vi "Sequencer Main.vi"() -> ()   [LabVIEW 2018] (continued)
                                frame True {
                                n2569 = Scan From String(format string="%d", input string=w5408, initial scan location=u32 1) -> (output 1=w5405:i32)  [unwired: 2 in, 3 out]
                                }
                                }
                                n2570 = In Range and Coerce(upper limit=w5398, x=w5395, lower limit=w5397) -> (In Range?=w5396:bool)  [unwired: 1 out]
                                }
                                }
                                n2571 = Replace Array Subset(array=w5392, new element=w5388, index=3) -> (w5391:errorcluster[])
                                n2572 = global write "Global Variable.vi" "Array Errors"(w5391) -> ()
                                n2573 = Number To Decimal String(number=w5383) -> (decimal integer string=w5371:string)  [unwired: 1 in]
                                n2574 = Concatenate Strings(w5378, "::") -> (w5379:string)
                                n2575 = Concatenate Strings(w5382, w5381, w5382, w5379, w5374, w5375, w5373, w5374, w5371, w5373, w5374, w5372, w5373, w5380, w5381, w5380) -> (w5376:string)
                                n2576 = case shown="False" w5384 {
                                tunnel: [enum16{"Idle", "PASS", "FALSE"}."FALSE" ("Step Test Result") enum16{"Idle", "PASS", "FALSE"}."PASS" ("Step Test Result")] -> w5389
                                frame False {
                                # "Step TEST Result"
                                }
                                frame True {
                                # "Step TEST Result"
                                }
                                }
                                n2577 = invoke on="Serial CMD Mon" class="Str" method="Append String"("string"=w5376) -> ()  [unwired: 3 in, 4 out]
                                }
                                frame #2 {
                                }
                              }
                              n2578 = global read "Global Variable.vi" "Array_Measurement"() -> (w5339:dbl[])
                              n2579 = Decimal String To Number(string=w5329) -> (number=w5340:i32)  [unwired: 2 in, 1 out]
                              n2580 = Index Array(array=w5339, index=w5340) -> (element=w5338:dbl)
                              n2581 = in-place {
                                in-place-border: w5338 -> [w5358]
                                in-place-border: [w5356] -> w5337
                                in-place-border: [w5353] -> w5336
                                w5354 = 1000.0 ("y")
                                # "Calculate +-3%"
                                n2582 = Multiply(x=w5358, y=1.03) -> (x*y=w5359:dbl)
                                n2583 = Multiply(x=w5358, y=0.97) -> (x*y=w5355:dbl)
                                n2584 = Multiply(x=w5359, y=w5354) -> (x*y=w5356:dbl)
                                n2585 = Multiply(x=w5354, y=w5355) -> (x*y=w5353:dbl)
                              }
                              n2586 = To Unsigned Long Integer(number=w5337) -> (unsigned 32bit integer=w5334:u32)
                              n2587 = To Unsigned Long Integer(number=w5336) -> (unsigned 32bit integer=w5335:u32)
                              n2588 = Number To Decimal String(number=w5334) -> (decimal integer string=w5332:string)  [unwired: 1 in]
                              n2589 = Number To Decimal String(number=w5335) -> (decimal integer string=w5330:string)  [unwired: 1 in]
                              n2590 = Concatenate Strings("max " ("string"), w5332) -> (w5324:string)
                              n2591 = Concatenate Strings("min " ("string"), w5330) -> (w5323:string)
                              n2592 = Concatenate Strings(w5324, "\r\n", w5323) -> (w5325:string)
                              n2593 = in-place {
                                in-place-border: w5327 -> [w5348]
                                in-place-border: w5325 -> [w5346]
                                # "Set Parameters to \nTest Seguenser Table"
                                n2594 = global read "Global Variable.vi" "Current Step Nmb"() -> (w5350:u32)
                                n2595 = property on="Test Squencer Edit" class="MCListbox (strict)"() -> ("ItemNames"=w5352:string[][])  [unwired: 2 in, 2 out]
                                n2596 = Replace Array Subset(array=w5352, new element #1=w5348, index (row) #1=w5350, index (col) #1=2 ("disabled index (col)"), new element #2=w5346, index (row) #2=w5350, index (col) #2=4 ("disabled index (col)")) -> (w5351:string[][])
                                n2597 = property on="Test Squencer Edit" class="MCListbox (strict)"("ItemNames"=w5351) -> ()  [unwired: 2 in, 2 out]
                              }
                            }
                            frame "capmem" {
                              w5419 = "max: "
                              w5420 = ">" ("string")
                              w5422 = "<" ("string")
                              w5424 = "min: "
                              # "Parameters"
                              # "Cmd"
                              n2598 = flat-sequence {
                                tunnel: [w5456] -> w5442
                                tunnel: [w5455] -> w5441
                                tunnel: [w5454] -> w5413
                                tunnel: w5442 -> [w5491]
                                tunnel: w5441 -> [w5492]
                                tunnel: w5438 -> [w5490]
                                tunnel: w5433 -> [w5489]
                                tunnel: w5437 -> [w5487]
                                tunnel: w5436 -> [w5486]
                                tunnel: [w5485] -> w5429
                                tunnel: [w5488] -> w5415
                                tunnel: [w5569] -> w5414
                                tunnel: w5415 -> [w5569]
                                frame #0 {
                                n2599 = for {
                                N: 1 -> [_]
                                tunnel: [w5461] -> w5456
                                tunnel: [w5460] -> w5455
                                tunnel: [w5458] -> w5454
                                i -> [w5459]
                                n2600 = case shown="1" w5459 {
                                tunnel: [w5467 w5481] -> w5461
                                tunnel: [w5463 w5474] -> w5460
                                tunnel: [w5462 w5473] -> w5458
                                frame 0, Default {
                                n2601 = global read "Global Variable.vi" "COM Port FTDI RS232"() -> (w5470:refnum<visa-resource-name>)
                                n2602 = call "ADB-Serial_WrRd.vi"("Timeout(Sec)"=2.0, "PassString"="Chuck(3)", "Command"="capmem 1", "ComPort"=w5470) -> ("error out"=w5464:errorcluster, "PASS"=w5467:bool, "received"=w5462:string)  [unwired: 5 in]
                                n2603 = invoke on="Serial CMD Mon" class="Str" method="Append String"(error in=w5464, "string"=w5462) -> (error out=w5463:errorcluster)  [unwired: 2 in, 3 out]
                                n2604 = Wait (ms)(milliseconds to wait=u32 1000) -> ()  [unwired: 1 out]
                                }
                                frame 1 {
                                w5471 = u16 2 items=["None", "XON/XOFF", "RTS/CTS", "XON/XOFF & RTS/CTS", "DTR/DSR", "XON/XOFF & DTR/DSR"] ("flow control (0:none)")
                                w5476 = "\r\n"
                                n2605 = global read "Global Variable.vi" "COM Port FTDI RS232"() -> (w5484:refnum<visa-resource-name>)
                                n2606 = call "ADB-Serial_WrRd.vi"("flow control (0:none)"=w5471, "Tx Deay"=u16 5, "Timeout(Sec)"=2.0, "PassString"="Chuck(3)", "Command"="capmem 0", "ComPort"=w5484) -> ("error out"=w5475:errorcluster, "PASS"=w5481:bool, "received"=w5473:string)  [unwired: 3 in]
                                n2607 = Concatenate Strings(w5473, w5476, "DELAY->5Sec", w5476) -> (w5478:string)
                                n2608 = invoke on="Serial CMD Mon" class="Str" method="Append String"(error in=w5475, "string"=w5478) -> (error out=w5474:errorcluster)  [unwired: 2 in, 3 out]
                                n2609 = Wait (ms)(milliseconds to wait=u32 4500) -> ()  [unwired: 1 out]
                                }
                                }
                                }
                                }
                                frame #1 {
                                n2610 = case shown="True" w5491 {
                                tunnel: w5490 -> [_ w5509]
                                tunnel: w5489 -> [_ w5508]
                                tunnel: [enum16{"Idle", "PASS", "FALSE"}."FALSE" ("Step Test Result") w5507] -> w5488
                                tunnel: w5487 -> [_ w5506]
                                tunnel: w5486 -> [_ w5505]
                                tunnel: [i32[] [0, 0] w5498] -> w5485
                                frame False {
                                }
                                frame True {
                                n2611 = for {
                                N: 2 -> [_]
                                tunnel: w5509 -> [w5518]
                                tunnel: w5508 -> [w5517]
                                tunnel: w5506 -> [w5516]
                                tunnel: w5505 -> [w5515]
                                tunnel: [w5514] -> w5504 mode=indexing
                                tunnel: [w5513] -> w5498 mode=indexing
                                i -> [w5519]
                                n2612 = case shown="1" w5519 {
                                tunnel: w5518 -> [w5534 _]
                                tunnel: w5517 -> [w5533 _]
                                tunnel: w5516 -> [_ w5553]
                                tunnel: w5515 -> [_ w5552]
                                tunnel: [w5527 w5551] -> w5514
                                tunnel: [w5520 w5547] -> w5513
                                frame 0, Default {
                                w5523 = "\r\n"
                                n2613 = global read "Global Variable.vi" "COM Port FTDI RS232"() -> (w5540:refnum<visa-resource-name>)
                                n2614 = Wait (ms)(milliseconds to wait=u32 4500) -> ()  [unwired: 1 out]
                                n2615 = call "ADB-Serial_WrRd.vi"("Timeout(Sec)"=3.0, "PassString"="Chuck(3)", "Command"="capmem", "ComPort"=w5540) -> ("error out"=w5522:errorcluster, "PASS"=w5528:bool, "received"=w5525:string)  [unwired: 5 in]
                                n2616 = property on="Msg Str" class="Str"("Text.Scroll Position"=inf) -> ()  [unwired: 2 in, 2 out]
                                n2617 = Match Pattern(string=w5525, regular expression="voltage") -> (after substring=w5538:string)  [unwired: 1 in, 3 out]
                                n2618 = Concatenate Strings(w5525, w5523, "DELAY->5Sec", w5523) -> (w5526:string)
                                n2619 = Scan From String(format string="%d", input string=w5538, initial scan location=u32 0) -> (output 1=w5520:i32)  [unwired: 2 in, 3 out]
                                n2620 = global read "Global Variable.vi" "Array Errors"() -> (w5530:errorcluster[])
                                n2621 = In Range and Coerce(upper limit=w5534, x=w5520, lower limit=w5533) -> (In Range?=w5529:bool)  [unwired: 1 out]
                                n2622 = invoke on="Serial CMD Mon" class="Str" method="Append String"(error in=w5522, "string"=w5526) -> (error out=w5521:errorcluster)  [unwired: 2 in, 3 out]
                                n2623 = Replace Array Subset(array=w5530, new element=w5521, index=3) -> (w5531:errorcluster[])
                                n2624 = And(x=w5529, y=w5528) -> (x .and. y?=w5527:bool)
                                n2625 = global write "Global Variable.vi" "Array Errors"(w5531) -> ()
                                }
                                frame 1 {
                                w5545 = u16 2 items=["None", "XON/XOFF", "RTS/CTS", "XON/XOFF & RTS/CTS", "DTR/DSR", "XON/XOFF & DTR/DSR"] ("flow control (0:none)")
                                n2626 = global read "Global Variable.vi" "COM Port FTDI RS232"() -> (w5564:refnum<visa-resource-name>)
                                n2627 = call "ADB-Serial_WrRd.vi"("flow control (0:none)"=w5545, "Tx Deay"=u16 5, "Timeout(Sec)"=3.0, "PassString"="Chuck(3)", "Command"="capmem", "ComPort"=w5564) -> ("error out"=w5549:errorcluster, "PASS"=w5554:bool, "received"=w5550:string)  [unwired: 3 in]
                                n2628 = invoke on="Serial CMD Mon" class="Str" method="Append String"("string"=w5550) -> ()  [unwired: 3 in, 4 out]
                                n2629 = property on="Msg Str" class="Str"(error in=w5549, "Text.Scroll Position"=inf) -> (error out=w5548:errorcluster)  [unwired: 1 in, 1 out]
                                n2630 = Match Pattern(string=w5550, regular expression="voltage") -> (after substring=w5562:string)  [unwired: 1 in, 3 out]
                                n2631 = Scan From String(format string="%d", input string=w5562, initial scan location=u32 0) -> (output 1=w5547:i32)  [unwired: 2 in, 3 out]
                                n2632 = global read "Global Variable.vi" "Array Errors"() -> (w5556:errorcluster[])
                                n2633 = In Range and Coerce(upper limit=w5553, x=w5547, lower limit=w5552) -> (In Range?=w5555:bool)  [unwired: 1 out]
                                n2634 = Replace Array Subset(array=w5556, new element=w5548, index=3) -> (w5557:errorcluster[])
                                n2635 = global write "Global Variable.vi" "Array Errors"(w5557) -> ()
                                n2636 = And(x=w5555, y=w5554) -> (x .and. y?=w5551:bool)
                                n2637 = Wait (ms)(milliseconds to wait=u32 1000) -> ()  [unwired: 1 out]
                                }
                                }
                                }
                                n2638 = Index Array(array=w5504, index #1=0 ("index"), index #2=1 ("index")) -> (element #1=w5503:bool, element #2=w5502:bool)
                                n2639 = And(x=w5503, y=w5502) -> (x .and. y?=w5501:bool)
                                n2640 = case shown="True" w5501 {
                                tunnel: [enum16{"Idle", "PASS", "FALSE"}."FALSE" ("Step Test Result") enum16{"Idle", "PASS", "FALSE"}."PASS" ("Step Test Result")] -> w5507
                                frame False {
                                # "Step TEST Result"
                                }
                                frame True {
                                # "Step TEST Result"
                                }
                                }
                                }
                                }
                                n2641 = global read "Global Variable.vi" "Array Errors"() -> (w5495:errorcluster[])
                                n2642 = Replace Array Subset(array=w5495, new element=w5492, index=3) -> (w5494:errorcluster[])
                                n2643 = global write "Global Variable.vi" "Array Errors"(w5494) -> ()
                                }
                                frame #2 {
                                }
                              }
                              n2644 = in-place {
                                in-place-border: w5440 -> [w5453]
                                in-place-border: w5439 -> [w5452]
                                in-place-border: [w5450] -> w5438
                                in-place-border: [w5449] -> w5433
                                in-place-border: [w5448] -> w5437
                                in-place-border: [w5447] -> w5436
                                in-place-border: [w5444] -> w5432
                                in-place-border: [w5443] -> w5426
                                in-place-border: [w5446] -> w5423
                                in-place-border: [w5445] -> w5418
                                w5451 = "-"
                                # "param-2 : min / max"
                                # "param-1 : min / max"
                                n2645 = Match Pattern(string=w5453, regular expression=w5451) -> (before substring=w5443:string, after substring=w5444:string)  [unwired: 1 in, 2 out]
                                n2646 = Match Pattern(string=w5452, regular expression=w5451) -> (before substring=w5445:string, after substring=w5446:string)  [unwired: 1 in, 2 out]
                                n2647 = Decimal String To Number(string=w5444) -> (number=w5449:i32)  [unwired: 2 in, 1 out]
                                n2648 = Decimal String To Number(string=w5446) -> (number=w5447:i32)  [unwired: 2 in, 1 out]
                                n2649 = Decimal String To Number(string=w5443) -> (number=w5450:i32)  [unwired: 2 in, 1 out]
                                n2650 = Decimal String To Number(string=w5445) -> (number=w5448:i32)  [unwired: 2 in, 1 out]
                              }
                              n2651 = Index Array(array=w5429, index #1=0, index #2=1) -> (element #1=w5417:i32, element #2=w5427:i32)
                              n2652 = Number To Decimal String(number=w5417) -> (decimal integer string=w5428:string)  [unwired: 1 in]
                              n2653 = Number To Decimal String(number=w5427) -> (decimal integer string=w5421:string)  [unwired: 1 in]
                              n2654 = Concatenate Strings("Delay-5S -> ", w5424, w5432, w5422, w5428, w5420, w5419, w5426, "\r\n", "Delay-5S -> ", w5424, w5423, w5422, w5421, w5420, w5419, w5418) -> (w5434:string)
                            }
                            frame "capmem_set" {
                              # "Need 2 Times!"
                              # "Parameters"
                              # "Cmd"
                              n2655 = flat-sequence {
                                tunnel: [w5584] -> w5575
                                tunnel: [w5583] -> w5574
                                tunnel: [w5576] -> w5570
                                tunnel: w5575 -> [w5613]
                                tunnel: w5574 -> [w5614]
                                tunnel: [w5612] -> w5573
                                tunnel: [w5611] -> w5571
                                tunnel: w5570 -> [w5611]
                                frame #0 {
                                w5577 = "\r\n"
                                n2656 = for {
                                N: 2 -> [_]
                                tunnel: [w5589] -> w5584
                                tunnel: [w5588] -> w5583
                                tunnel: [w5586] -> w5582 mode=indexing
                                i -> [w5587]
                                n2657 = case shown="1" w5587 {
                                tunnel: [w5595 w5607] -> w5589
                                tunnel: [w5591 w5602] -> w5588
                                tunnel: [w5590 w5601] -> w5586
                                frame 0, Default {
                                n2658 = global read "Global Variable.vi" "COM Port FTDI RS232"() -> (w5598:refnum<visa-resource-name>)
                                n2659 = call "ADB-Serial_WrRd.vi"("Timeout(Sec)"=1.0, "PassString"="Chuck(3)", "Command"="capmem 1", "ComPort"=w5598) -> ("error out"=w5592:errorcluster, "PASS"=w5595:bool, "received"=w5590:string)  [unwired: 5 in]
                                n2660 = invoke on="Serial CMD Mon" class="Str" method="Append String"(error in=w5592, "string"=w5590) -> (error out=w5591:errorcluster)  [unwired: 2 in, 3 out]
                                n2661 = Wait (ms)(milliseconds to wait=u32 1000) -> ()  [unwired: 1 out]
                                }
                                frame 1 {
                                w5599 = u16 2 items=["None", "XON/XOFF", "RTS/CTS", "XON/XOFF & RTS/CTS", "DTR/DSR", "XON/XOFF & DTR/DSR"] ("flow control (0:none)")
                                n2662 = global read "Global Variable.vi" "COM Port FTDI RS232"() -> (w5610:refnum<visa-resource-name>)
                                n2663 = call "ADB-Serial_WrRd.vi"("flow control (0:none)"=w5599, "Tx Deay"=u16 0, "Timeout(Sec)"=2.0, "PassString"="Chuck(3)", "Command"="capmem 0", "ComPort"=w5610) -> ("error out"=w5603:errorcluster, "PASS"=w5607:bool, "received"=w5601:string)  [unwired: 3 in]
                                n2664 = Concatenate Strings(w5601, "\r\n") -> (w5605:string)
                                n2665 = invoke on="Serial CMD Mon" class="Str" method="Append String"(error in=w5603, "string"=w5605) -> (error out=w5602:errorcluster)  [unwired: 2 in, 3 out]
                                }
                                }
                                }
                                n2666 = Index Array(array=w5582, index #1=0 ("index"), index #2=1 ("index")) -> (element #1=w5579:string, element #2=w5578:string)
                                n2667 = Concatenate Strings(w5579, w5577, w5578, w5577) -> (w5576:string)
                                }
                                frame #1 {
                                n2668 = case shown="True" w5613 {
                                tunnel: [enum16{"Idle", "PASS", "FALSE"}."FALSE" ("Step Test Result") enum16{"Idle", "PASS", "FALSE"}."PASS" ("Step Test Result")] -> w5612
                                frame False {
                                }
                                frame True {
                                # "Step TEST Result"
                                }
                                }
                                n2669 = global read "Global Variable.vi" "Array Errors"() -> (w5617:errorcluster[])
                                n2670 = Replace Array Subset(array=w5617, new element=w5614, index=3) -> (w5616:errorcluster[])
                                n2671 = global write "Global Variable.vi" "Array Errors"(w5616) -> ()
                                }
                              }
                            }
                            frame "capmem_get" {
                              # "Parameters"
                              # "Cmd"
                              n2672 = To Word Integer(number=w5628) -> (16bit integer=w5627:i16)
                              n2673 = To Word Integer(number=w5629) -> (16bit integer=w5626:i16)
                              n2674 = flat-sequence {
                                tunnel: [w5640] -> w5632
                                tunnel: [w5638] -> w5631
                                tunnel: [w5639] -> w5630
                                tunnel: w5632 -> [w5653]
                                tunnel: w5631 -> [w5652]
                                tunnel: w5630 -> [w5647]
                                tunnel: w5626 -> [w5651]
                                tunnel: w5627 -> [w5650]
                                tunnel: [w5649] -> w5625
                                tunnel: [w5648] -> w5624
                                tunnel: [w5646] -> w5621
                                tunnel: [w5645] -> w5620
                                frame #0 {
                                w5636 = u16 2 items=["None", "XON/XOFF", "RTS/CTS", "XON/XOFF & RTS/CTS", "DTR/DSR", "XON/XOFF & DTR/DSR"] ("flow control (0:none)")
                                n2675 = global read "Global Variable.vi" "COM Port FTDI RS232"() -> (w5641:refnum<visa-resource-name>)
                                n2676 = call "ADB-Serial_WrRd.vi"("flow control (0:none)"=w5636, "Tx Deay"=u16 5, "Timeout(Sec)"=2.0, "PassString"="Chuck(3)", "Command"="capmem", "ComPort"=w5641) -> ("error out"=w5639:errorcluster, "PASS"=w5640:bool, "received"=w5638:string)  [unwired: 3 in]
                                }
                                frame #1 {
                                n2677 = case shown="False" w5653 {
                                tunnel: w5652 -> [w5654 w5658]
                                tunnel: w5651 -> [_ w5663]
                                tunnel: w5650 -> [_ w5662]
                                tunnel: [FALSE w5661] -> w5649
                                tunnel: [w5656 w5660] -> w5648
                                tunnel: w5647 -> [w5656 w5660]
                                tunnel: [-1 w5659] -> w5646
                                tunnel: [w5654 w5658] -> w5645
                                frame False {
                                }
                                frame True {
                                n2678 = invoke on="Serial CMD Mon" class="Str" method="Append String"("string"=w5658) -> ()  [unwired: 3 in, 4 out]
                                n2679 = Match Pattern(string=w5658, regular expression="voltage") -> (after substring=w5667:string)  [unwired: 1 in, 3 out]
                                n2680 = Scan From String(format string="%d", input string=w5667, initial scan location=u32 0) -> (output 1=w5659:i32)  [unwired: 2 in, 3 out]
                                n2681 = In Range and Coerce(upper limit=w5663, x=w5659, lower limit=w5662) -> (In Range?=w5661:bool)  [unwired: 1 out]
                                }
                                }
                                }
                              }
                              n2682 = global read "Global Variable.vi" "Array Errors"() -> (w5633:errorcluster[])
                              n2683 = Replace Array Subset(array=w5633, new element=w5624, index=3) -> (w5634:errorcluster[])
                              n2684 = global write "Global Variable.vi" "Array Errors"(w5634) -> ()
                              n2685 = case shown="True" w5625 {
                                tunnel: [enum16{"Idle", "PASS", "FALSE"}."FALSE" ("Step Test Result") enum16{"Idle", "PASS", "FALSE"}."PASS" ("Step Test Result")] -> w5623
                                frame False {
                                # "Step TEST Result"
                                }
                                frame True {
                                # "Step TEST Result"
                                }
                              }
                              n2686 = Number To Decimal String(number=w5621) -> (decimal integer string=w5622:string)  [unwired: 1 in]
                            }
                            frame "setPowerRes" {
                              # "Param"
                              # "Cmd"
                              n2687 = flat-sequence {
                                tunnel: [w5681] -> w5676
                                tunnel: [w5680] -> w5675
                                tunnel: [w5679] -> w5674
                                tunnel: w5673 -> [w5678]
                                tunnel: w5676 -> [w5700]
                                tunnel: w5675 -> [w5701]
                                tunnel: [w5697] -> w5672
                                tunnel: w5674 -> [w5695]
                                tunnel: [w5696] -> w5671
                                tunnel: [w5695] -> w5670
                                frame #0 {
                                n2688 = for {
                                N: 1 -> [_]
                                tunnel: [w5685] -> w5681
                                tunnel: [w5694] -> w5680
                                shift-right: [w5684] -> w5679
                                shift-left: w5678 -> [w5689]
                                stop <- w5685 stop-if-true
                                w5682 = u16 2 items=["None", "XON/XOFF", "RTS/CTS", "XON/XOFF & RTS/CTS", "DTR/DSR", "XON/XOFF & DTR/DSR"] ("flow control (0:none)")
                                n2689 = call <vilib>:"Space Constant.vi"() -> ("String"=w5688:string)
                                n2690 = global read "Global Variable.vi" "COM Port FTDI RS232"() -> (w5693:refnum<visa-resource-name>)
                                n2691 = Concatenate Strings("setPowerRes", w5688, w5689) -> (w5687:string)
                                n2692 = call "ADB-Serial_WrRd.vi"("flow control (0:none)"=w5682, "Tx Deay"=u16 5, "Timeout(Sec)"=2.0, "PassString"="Set power resistor", "Command"=w5687, "ComPort"=w5693) -> ("error out"=w5694:errorcluster, "PASS"=w5685:bool, "received"=w5684:string)  [unwired: 3 in]
                                n2693 = invoke on="Serial CMD Mon" class="Str" method="Append String"("string"=w5684) -> ()  [unwired: 3 in, 4 out]
                                n2694 = Wait (ms)(milliseconds to wait=u32 500) -> ()  [unwired: 1 out]
                                }
                                }
                                frame #1 {
                                n2695 = global read "Global Variable.vi" "Array Errors"() -> (w5704:errorcluster[])
                                n2696 = call <userlib>:"Multi-line String to Array__ogtk.vi"("string"=w5695) -> ("lines"=w5699:string[])
                                n2697 = case shown="False" w5700 {
                                tunnel: [enum16{"Idle", "PASS", "FALSE"}."FALSE" ("Step Test Result") enum16{"Idle", "PASS", "FALSE"}."PASS" ("Step Test Result")] -> w5697
                                frame False {
                                # "Step TEST Result"
                                }
                                frame True {
                                # "Step TEST Result"
                                }
                                }
                                n2698 = Replace Array Subset(array=w5704, new element=w5701, index=3) -> (w5703:errorcluster[])
                                n2699 = Index Array(array=w5699, index=2 ("line index")) -> (element=w5696:string)
                                n2700 = global write "Global Variable.vi" "Array Errors"(w5703) -> ()
                                }
                              }
                            }
                            frame "calibADCoffset" {
                              # "Param"
                              # "Cmd"
                              n2701 = flat-sequence {
                                tunnel: [w5715] -> w5711
                                tunnel: [w5714] -> w5710
                                tunnel: [w5712] -> w5709
                                tunnel: w5711 -> [w5729]
                                tunnel: w5710 -> [w5730]
                                tunnel: [w5731] -> w5708
                                tunnel: w5709 -> [w5727]
                                tunnel: [w5727] -> w5707
                                frame #0 {
                                n2702 = for {
                                N: 1 -> [_]
                                tunnel: [w5721] -> w5715
                                tunnel: [w5726] -> w5714
                                tunnel: [w5718] -> w5712
                                stop <- w5721 stop-if-true
                                w5716 = u16 2 items=["None", "XON/XOFF", "RTS/CTS", "XON/XOFF & RTS/CTS", "DTR/DSR", "XON/XOFF & DTR/DSR"] ("flow control (0:none)")
                                n2703 = global read "Global Variable.vi" "COM Port FTDI RS232"() -> (w5725:refnum<visa-resource-name>)
                                n2704 = global write "Global Variable.vi" "ADC Offset"(0 ("ADC Offset")) -> ()
                                n2705 = call "ADB-Serial_WrRd.vi"("flow control (0:none)"=w5716, "Tx Deay"=u16 5, "Timeout(Sec)"=2.0, "PassString"="Chuck(3)", "Command"="calibADCoffset", "ComPort"=w5725) -> ("error out"=w5726:errorcluster, "PASS"=w5721:bool, "received"=w5718:string)  [unwired: 3 in]
                                n2706 = invoke on="Serial CMD Mon" class="Str" method="Append String"("string"=w5718) -> ()  [unwired: 3 in, 4 out]
                                n2707 = Wait (ms)(milliseconds to wait=u32 200) -> ()  [unwired: 1 out]
                                }
                                }
                                frame #1 {
                                n2708 = case shown="True" w5729 {
                                tunnel: w5727 -> [_ w5741]
                                tunnel: [FALSE w5736] -> w5728
                                frame False {
                                }
                                frame True {
                                n2709 = Match Pattern(string=w5741, regular expression="New ADC offset:") -> (after substring=w5739:string)  [unwired: 1 in, 3 out]
                                n2710 = Scan From String(format string="%d", input string=w5739) -> (output 1=w5737:i32)  [unwired: 3 in, 3 out]
                                n2711 = global write "Global Variable.vi" "ADC Offset"(w5737) -> ()
                                n2712 = Greater Than 0?(x=w5737) -> (x > 0?=w5736:bool)
                                }
                                }
                                n2713 = global read "Global Variable.vi" "Array Errors"() -> (w5734:errorcluster[])
                                n2714 = Replace Array Subset(array=w5734, new element=w5730, index=3) -> (w5733:errorcluster[])
                                n2715 = case shown="False" w5728 {
                                tunnel: [enum16{"Idle", "PASS", "FALSE"}."FALSE" ("Step Test Result") enum16{"Idle", "PASS", "FALSE"}."PASS" ("Step Test Result")] -> w5731
                                frame False {
                                # "Step TEST Result"
                                }
                                frame True {
                                # "Step TEST Result"
                                }
                                }
                                n2716 = global write "Global Variable.vi" "Array Errors"(w5733) -> ()
                                }
                              }
                            }
                            frame "calibCCRsave" {
                              # "Param"
                              # "Cmd"
                              n2717 = flat-sequence {
                                tunnel: [w5753] -> w5748
                                tunnel: [w5752] -> w5747
                                tunnel: w5746 -> [w5750]
                                tunnel: [w5749] -> w5744
                                tunnel: w5748 -> [w5769]
                                tunnel: w5747 -> [w5770]
                                tunnel: [w5767] -> w5745
                                frame #0 {
                                n2718 = for {
                                N: 1 -> [_]
                                tunnel: [w5761] -> w5753
                                tunnel: [w5766] -> w5752
                                tunnel: w5750 -> [w5758]
                                tunnel: [w5757] -> w5749
                                stop <- w5761 stop-if-true
                                w5754 = u16 2 items=["None", "XON/XOFF", "RTS/CTS", "XON/XOFF & RTS/CTS", "DTR/DSR", "XON/XOFF & DTR/DSR"] ("flow control (0:none)")
                                (unwired) ""
                                n2719 = global read "Global Variable.vi" "COM Port FTDI RS232"() -> (w5765:refnum<visa-resource-name>)
                                n2720 = call <vilib>:"Space Constant.vi"() -> ("String"=w5756:string)
                                n2721 = Concatenate Strings("calibCCRsave", w5756, w5758) -> (w5759:string)
                                n2722 = call "ADB-Serial_WrRd.vi"("flow control (0:none)"=w5754, "Tx Deay"=u16 0, "Timeout(Sec)"=2.0, "PassString"="Chuck(3)", "Command"=w5759, "ComPort"=w5765) -> ("error out"=w5766:errorcluster, "PASS"=w5761:bool, "received"=w5757:string)  [unwired: 3 in]
                                n2723 = invoke on="Serial CMD Mon" class="Str" method="Append String"("string"=w5757) -> ()  [unwired: 3 in, 4 out]
                                n2724 = Wait (ms)(milliseconds to wait=u32 200) -> ()  [unwired: 1 out]
                                }
                                }
                                frame #1 {
                                n2725 = global read "Global Variable.vi" "Array Errors"() -> (w5773:errorcluster[])
                                n2726 = case shown="True" w5769 {
                                tunnel: [FALSE w5775] -> w5768
                                frame False {
                                }
                                frame True {
                                n2727 = global read "Global Variable.vi" "ADC Offset"() -> (w5776:i32)
                                n2728 = Greater Than 0?(x=w5776) -> (x > 0?=w5775:bool)
                                }
                                }
                                n2729 = Replace Array Subset(array=w5773, new element=w5770, index=3) -> (w5772:errorcluster[])
                                n2730 = global write "Global Variable.vi" "Array Errors"(w5772) -> ()
                                n2731 = case shown="False" w5768 {
                                tunnel: [enum16{"Idle", "PASS", "FALSE"}."FALSE" ("Step Test Result") enum16{"Idle", "PASS", "FALSE"}."PASS" ("Step Test Result")] -> w5767
                                frame False {
                                # "Step TEST Result"
                                }
                                frame True {
                                # "Step TEST Result"
                                }
                                }
                                }
                              }
                            }
                            frame "start_ble" {
                              # "Param"
                              # "Cmd"
                              n2732 = flat-sequence {
                                tunnel: [w5788] -> w5784
                                tunnel: [w5787] -> w5783
                                tunnel: [w5785] -> w5781
                                tunnel: [w5785] -> w5779
                                tunnel: w5784 -> [w5803]
                                tunnel: w5783 -> [w5804]
                                tunnel: [w5805] -> w5782
                                tunnel: w5781 -> [w5802]
                                tunnel: [w5800] -> w5780
                                frame #0 {
                                n2733 = for {
                                N: 1 -> [_]
                                tunnel: [w5793] -> w5788
                                tunnel: [w5798] -> w5787
                                tunnel: [w5791] -> w5785
                                stop <- w5793 stop-if-true
                                w5789 = u16 2 items=["None", "XON/XOFF", "RTS/CTS", "XON/XOFF & RTS/CTS", "DTR/DSR", "XON/XOFF & DTR/DSR"] ("flow control (0:none)")
                                n2734 = global read "Global Variable.vi" "COM Port FTDI RS232"() -> (w5797:refnum<visa-resource-name>)
                                n2735 = call "ADB-Serial_WrRd.vi"("flow control (0:none)"=w5789, "Tx Deay"=u16 5, "Timeout(Sec)"=7.0, "PassString"="Chuck(3)", "Command"="start_ble", "ComPort"=w5797) -> ("error out"=w5798:errorcluster, "PASS"=w5793:bool, "received"=w5791:string)  [unwired: 3 in]
                                n2736 = invoke on="Serial CMD Mon" class="Str" method="Append String"("string"=w5791) -> ()  [unwired: 3 in, 4 out]
                                n2737 = Wait (ms)(milliseconds to wait=u32 200) -> ()  [unwired: 1 out]
                                }
                                }
                                frame #1 {
                                n2738 = global read "Global Variable.vi" "Array Errors"() -> (w5808:errorcluster[])
                                n2739 = call <userlib>:"Multi-line String to Array__ogtk.vi"("string"=w5802) -> ("lines"=w5801:string[])
                                n2740 = Index Array(array=w5801, index=4) -> (element=w5800:string)
                                n2741 = Replace Array Subset(array=w5808, new element=w5804, index=3) -> (w5807:errorcluster[])
                                n2742 = global write "Global Variable.vi" "Array Errors"(w5807) -> ()
                                n2743 = case shown="False" w5803 {
                                tunnel: [enum16{"Idle", "PASS", "FALSE"}."FALSE" ("Step Test Result") enum16{"Idle", "PASS", "FALSE"}."PASS" ("Step Test Result")] -> w5805
                                frame False {
                                # "Step TEST Result"
                                }
                                frame True {
                                # "Step TEST Result"
                                }
                                }
                                }
                              }
                            }
                            frame "enable_ble" {
                              # "Param"
                              # "Cmd"
                              n2744 = flat-sequence {
                                tunnel: [w5820] -> w5816
                                tunnel: [w5819] -> w5815
                                tunnel: [w5817] -> w5813
                                tunnel: [w5817] -> w5811
                                tunnel: w5816 -> [w5835]
                                tunnel: w5815 -> [w5836]
                                tunnel: [w5837] -> w5814
                                tunnel: w5813 -> [w5834]
                                tunnel: [w5832] -> w5812
                                frame #0 {
                                n2745 = for {
                                N: 1 -> [_]
                                tunnel: [w5825] -> w5820
                                tunnel: [w5830] -> w5819
                                tunnel: [w5823] -> w5817
                                stop <- w5825 stop-if-true
                                w5821 = u16 2 items=["None", "XON/XOFF", "RTS/CTS", "XON/XOFF & RTS/CTS", "DTR/DSR", "XON/XOFF & DTR/DSR"] ("flow control (0:none)")
                                n2746 = global read "Global Variable.vi" "COM Port FTDI RS232"() -> (w5829:refnum<visa-resource-name>)
                                n2747 = call "ADB-Serial_WrRd.vi"("flow control (0:none)"=w5821, "Tx Deay"=u16 5, "Timeout(Sec)"=7.0, "PassString"="Chuck(3)", "Command"="enable_ble", "ComPort"=w5829) -> ("error out"=w5830:errorcluster, "PASS"=w5825:bool, "received"=w5823:string)  [unwired: 3 in]
                                n2748 = invoke on="Serial CMD Mon" class="Str" method="Append String"("string"=w5823) -> ()  [unwired: 3 in, 4 out]
                                n2749 = Wait (ms)(milliseconds to wait=u32 200) -> ()  [unwired: 1 out]
                                }
                                }
                                frame #1 {
                                n2750 = global read "Global Variable.vi" "Array Errors"() -> (w5840:errorcluster[])
                                n2751 = call <userlib>:"Multi-line String to Array__ogtk.vi"("string"=w5834) -> ("lines"=w5833:string[])
                                n2752 = Index Array(array=w5833, index=4) -> (element=w5832:string)
                                n2753 = Replace Array Subset(array=w5840, new element=w5836, index=3) -> (w5839:errorcluster[])
                                n2754 = global write "Global Variable.vi" "Array Errors"(w5839) -> ()
                                n2755 = case shown="False" w5835 {
                                tunnel: [enum16{"Idle", "PASS", "FALSE"}."FALSE" ("Step Test Result") enum16{"Idle", "PASS", "FALSE"}."PASS" ("Step Test Result")] -> w5837
                                frame False {
                                # "Step TEST Result"
                                }
                                frame True {
                                # "Step TEST Result"
                                }
                                }
                                }
                              }
                            }
                            frame "setopvg" {
                              # "Param"
                              # "Cmd"
                              n2756 = flat-sequence {
                                tunnel: [w5853] -> w5848
                                tunnel: [w5852] -> w5847
                                tunnel: [w5850] -> w5845
                                tunnel: w5844 -> [w5849]
                                tunnel: w5848 -> [w5868]
                                tunnel: w5847 -> [w5869]
                                tunnel: [w5870] -> w5846
                                tunnel: w5845 -> [w5867]
                                tunnel: [w5867] -> w5843
                                frame #0 {
                                n2757 = for {
                                N: 1 -> [_]
                                tunnel: [w5861] -> w5853
                                tunnel: [w5866] -> w5852
                                tunnel: [w5856] -> w5850
                                tunnel: w5849 -> [w5858]
                                stop <- w5861 stop-if-true
                                w5854 = u16 2 items=["None", "XON/XOFF", "RTS/CTS", "XON/XOFF & RTS/CTS", "DTR/DSR", "XON/XOFF & DTR/DSR"] ("flow control (0:none)")
                                n2758 = global read "Global Variable.vi" "COM Port FTDI RS232"() -> (w5865:refnum<visa-resource-name>)
                                n2759 = call <vilib>:"Space Constant.vi"() -> ("String"=w5859:string)
                                n2760 = Concatenate Strings("setopvg", w5859, w5858) -> (w5857:string)
                                n2761 = call "ADB-Serial_WrRd.vi"("flow control (0:none)"=w5854, "Tx Deay"=u16 5, "Timeout(Sec)"=2.0, "PassString"="Chuck(3)", "Command"=w5857, "ComPort"=w5865) -> ("error out"=w5866:errorcluster, "PASS"=w5861:bool, "received"=w5856:string)  [unwired: 3 in]
                                n2762 = invoke on="Serial CMD Mon" class="Str" method="Append String"("string"=w5856) -> ()  [unwired: 3 in, 4 out]
                                n2763 = Wait (ms)(milliseconds to wait=u32 200) -> ()  [unwired: 1 out]
                                }
                                }
                                frame #1 {
                                n2764 = global read "Global Variable.vi" "Array Errors"() -> (w5873:errorcluster[])
                                n2765 = case shown="True" w5868 {
                                tunnel: [enum16{"Idle", "PASS", "FALSE"}."FALSE" ("Step Test Result") enum16{"Idle", "PASS", "FALSE"}."PASS" ("Step Test Result")] -> w5870
                                frame False {
                                # "Step TEST Result"
                                }
                                frame True {
                                # "Step TEST Result"
                                }
                                }
                                n2766 = Replace Array Subset(array=w5873, new element=w5869, index=3) -> (w5872:errorcluster[])
                                n2767 = global write "Global Variable.vi" "Array Errors"(w5872) -> ()
                                }
                              }
                            }
                            frame "reset" {
                              # "Param"
                              # "Cmd"
                              n2768 = flat-sequence {
                                tunnel: [w5884] -> w5880
                                tunnel: [w5883] -> w5879
                                tunnel: [w5881] -> w5876
                                tunnel: w5880 -> [w5896]
                                tunnel: w5879 -> [w5897]
                                tunnel: [w5898] -> w5878
                                tunnel: [w5895] -> w5877
                                tunnel: w5876 -> [w5895]
                                frame #0 {
                                n2769 = for {
                                N: 1 -> [_]
                                tunnel: [w5890] -> w5884
                                tunnel: [w5894] -> w5883
                                tunnel: [w5887] -> w5881
                                stop <- w5890 stop-if-true
                                w5885 = u16 2 items=["None", "XON/XOFF", "RTS/CTS", "XON/XOFF & RTS/CTS", "DTR/DSR", "XON/XOFF & DTR/DSR"] ("flow control (0:none)")
                                n2770 = global read "Global Variable.vi" "COM Port FTDI RS232"() -> (w5893:refnum<visa-resource-name>)
                                n2771 = call "ADB-Serial_WrRd.vi"("flow control (0:none)"=w5885, "Tx Deay"=u16 5, "Timeout(Sec)"=2.0, "PassString"="", "Command"="reset", "ComPort"=w5893) -> ("error out"=w5894:errorcluster, "PASS"=w5890:bool, "received"=w5887:string)  [unwired: 3 in]
                                n2772 = invoke on="Serial CMD Mon" class="Str" method="Append String"("string"=w5887) -> ()  [unwired: 3 in, 4 out]
                                n2773 = Wait (ms)(milliseconds to wait=u32 500) -> ()  [unwired: 1 out]
                                }
                                }
                                frame #1 {
                                n2774 = global read "Global Variable.vi" "Array Errors"() -> (w5901:errorcluster[])
                                n2775 = case shown="True" w5896 {
                                tunnel: [enum16{"Idle", "PASS", "FALSE"}."FALSE" ("Step Test Result") enum16{"Idle", "PASS", "FALSE"}."PASS" ("Step Test Result")] -> w5898
                                frame False {
                                # "Step TEST Result"
                                }
                                frame True {
                                # "Step TEST Result"
                                }
                                }
                                n2776 = Replace Array Subset(array=w5901, new element=w5897, index=3) -> (w5900:errorcluster[])
                                n2777 = global write "Global Variable.vi" "Array Errors"(w5900) -> ()
                                }
                              }
                            }
                          }
                          n2778 = local read "Debugging"() -> (w4690:bool)
                          n2779 = in-place {
                            in-place-border: w4691 -> [w4734]
                            in-place-border: [w4733] -> w4687
                            in-place-border: [w4732] -> w4688
                            # "GoTo Test-nmb"
                            # "ReTest Cyckles"
                            n2780 = Index Array(array=w4734, index #1=0, index #2=1, index #3=2) -> (element #2=w4738:string, element #3=w4739:string)  [unwired: 1 out]
                            n2781 = Decimal String To Number(string=w4738) -> (number=w4733:i32)  [unwired: 2 in, 1 out]
                            n2782 = Decimal String To Number(string=w4739) -> (number=w4732:i32)  [unwired: 2 in, 1 out]
                          }
                          n2783 = case shown="False" w4690 {
                            tunnel: w4689 -> [w4719 _]
                            tunnel: w4687 -> [w4717 _]
                            tunnel: w4688 -> [w4716 _]
                            frame False {
                              # "No Debug Mode"
                              n2784 = in-place {
                                in-place-border: [w4721] -> w4718
                                n2785 = global read "Global Variable.vi" "Retest Cnt"() -> (w4722:i16)
                                n2786 = Equal?(x=w4722, y=i16 0) -> (x = y?=w4721:bool)
                              }
                              n2787 = case shown="True" w4719 {
                                tunnel: w4718 -> [_ w4726]
                                tunnel: w4717 -> [_ w4724]
                                tunnel: w4716 -> [_ w4723]
                                frame False {
                                }
                                frame True {
                                # "String \"false\" Present"
                                n2788 = global write "Global Variable.vi" "Retest Step Nmb"(w4724) -> ()
                                n2789 = global write "Global Variable.vi" "Retest Nmb"(w4723) -> ()
                                n2790 = case shown="False" w4726 {
                                tunnel: w4723 -> [_ w4731]
                                frame False {
                                n2791 = global read "Global Variable.vi" "Retest Cnt"() -> (w4729:i16)
                                n2792 = Decrement(x=w4729) -> (x-1=w4728:i16)
                                n2793 = global write "Global Variable.vi" "Retest Cnt"(w4728) -> ()
                                n2794 = Wait (ms)(milliseconds to wait=u32 1000) -> ()  [unwired: 1 out]
                                }
                                frame True {
                                # "if(Retest-OFF & Cnt=0)"
                                n2795 = Decrement(x=w4731) -> (x-1=w4730:i32)
                                n2796 = global write "Global Variable.vi" "Retest Cnt"(w4730) -> ()
                                }
                                }
                                n2797 = global write "Global Variable.vi" "Retest ON"(TRUE ("Retest ON")) -> ()
                                }
                              }
                            }
                            frame True {
                            }
                          }
                          n2798 = in-place {
                            in-place-border: w4681 -> [w4713]
                            in-place-border: w4682 -> [w4712]
                            in-place-border: w4683 -> [w4711]
                            n2799 = call "Log Add Msg.vi"("Result"=w4711, "Communication"=w4712, "Description"=w4713) -> ("Out Msg"=w4714:string)
                            n2800 = property on="LogMsg" class="Str"("Text.Scroll Position"=inf) -> ()  [unwired: 2 in, 2 out]
                            n2801 = invoke on="LogMsg" class="Str" method="Append String"("string"=w4714) -> ()  [unwired: 3 in, 4 out]
                          }
                        }
                        frame 70 {
                          w5911 = "\r\n"
                          # "Step TEST Result"
                          # "FLASH Case"
                          # "FLASH Case"
                          n2802 = Unbundle By Name(w5916) -> ("Step Description"=w5906:string, "Parameters"=w5912:string)  [unwired: 1 out]
                          n2803 = Concatenate Strings("FLASH ADB Board", w5911, w5912, w5911) -> (w5910:string)
                          n2804 = invoke on="Msg Str" class="Str" method="Append String"("string"=w5910) -> (error out=w5909:errorcluster)  [unwired: 3 in, 3 out]
                          n2805 = property on="Tab Control Msg" class="TabCtl (strict)"("Value"=T21."Msg" ("Tab Control Msg")) -> (error out=w5914:errorcluster)  [unwired: 2 in, 1 out]
                          n2806 = in-place {
                            in-place-border: w5914 -> [_]
                            in-place-border: w5912 -> [w5932]
                            in-place-border: w5909 -> [_]
                            in-place-border: [w5927] -> w5908
                            in-place-border: [w5926] -> w5905
                            n2807 = call "Flash_ADB.vi"("Flash Bat File"=w5932) -> ("error out"=w5928:errorcluster, "standard output"=w5926:string, "Result"=w5927:bool)  [unwired: 7 in, 1 out]
                            n2808 = global read "Global Variable.vi" "Array Errors"() -> (w5930:errorcluster[])
                            n2809 = invoke on="Msg Str" class="Str" method="Append String"("string"=w5926) -> ()  [unwired: 3 in, 4 out]
